vi "Untitled 1.vi"   [LabVIEW 2021]
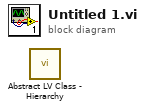
[diagram p0: block diagram]
diagram:
  n1 = call <vilib>:"Abstract LV Class - Hierarchy.vi"() -> ()  [unwired: 12 in]
